vi "Build New Ballard ARINC 429 Custom Device.vi"() -> ()   [LabVIEW 2020, in "Ballard ARINC 429 Scripting Examples.lvlib"]
uses:
  Ballard ARINC 429 Scripting Examples.lvlib
  <vilib>/addons/VeriStand Custom Device Scripting APIs/Ballard ARINC 429/Custom Device Support/Shared/Direction.ctl
  <vilib>/addons/VeriStand Custom Device Scripting APIs/Ballard ARINC 429/Custom Device Support/Shared/SDI.ctl
  <vilib>/addons/VeriStand Custom Device Scripting APIs/Ballard ARINC 429/Custom Device Support/Shared/Transfer Type.ctl
  <vilib>/addons/VeriStand Custom Device Scripting APIs/Ballard ARINC 429/Custom Device Support/Shared/Parameter Definition.ctl
  <vilib>/addons/VeriStand Custom Device Scripting APIs/Ballard ARINC 429/Encoding and Decoding/Encoding.ctl
  NationalInstruments.VeriStand.SystemDefinitionAPI
  niveristand-routing-and-faulting-custom-device/Source/Scripting Examples/SLSC Switch Examples.lvlib
  <vilib>/addons/VeriStand Custom Device Scripting APIs/Ballard ARINC 429/Custom Device Support/Scripting/Ballard/Ballard ARINC 429 Scripting.lvlib
  <vilib>/addons/VeriStand Custom Device Scripting APIs/Ballard ARINC 429/Encoding and Decoding/Encoding and Decoding.lvlib
panel:
  in  "Base System Definition File":path=path "Support/Base.nivssdf"
  in  "Output System Definition File":path=path "Support/Scripted Ballard ARINC 429.nivssdf"
  in  "Hardware Configuration File":path=path "Support/HW_Rx00_Tx24_Scheduled and Dynamic Labels.xml"
  # "Overview: Demonstrates using the Ballard ARINC 429 scripting API to configure the custom device by building from configuration clusters. \n\nInstructions:\n1. Specify the Hardware Configuration File. The hardware configuration file must be consistent with the schema installed by the Ballard hardware driver at C:\\Program Files (x86)\\Astronics Ballard Technology LabVIEW Driver\\Help\\index.html. The hardware configuration file must also be consistent with the configuration in this example VI.\n2. (VeriStand) Optionally, you may open the Output System Definition File in VeriStand, configure the Target, and deploy the scripted system definition to perform avionics bus communications with Ballard ARINC 429 hardware."
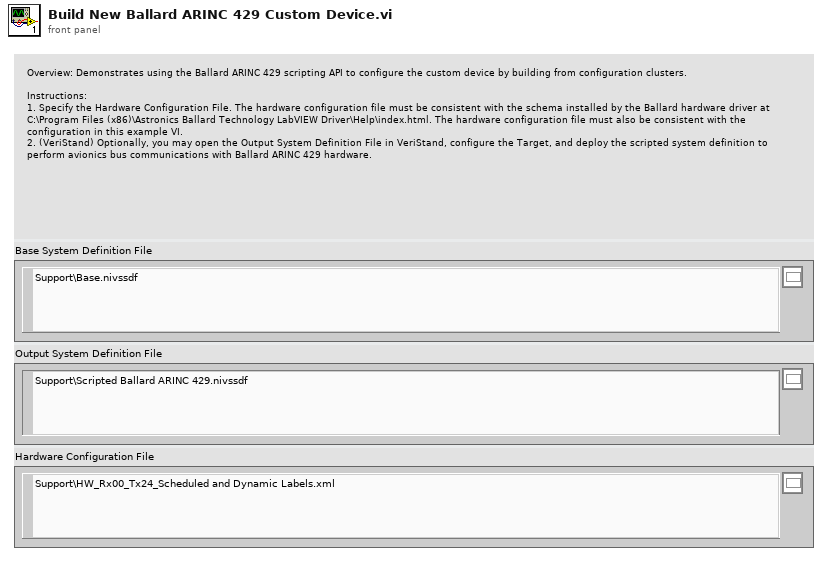
[diagram p1: front panel]
types:
  T1 = cluster{"name":string, "unit":string, "default value":dbl}[]
  T2 = typedef "Parameter Definition.ctl" = cluster{"start index":i32, "size":i32, "encoding":T3, "signed":bool, "scale multiplier":dbl, "scale offset":dbl}
  T3 = typedef "Encoding and Decoding.lvlib/Encoding.ctl" = enum16{"BNR", "BCD", "Discrete"}
  T4 = typedef "Direction.ctl" = enum16{"Rx", "Tx"}
  T5 = typedef "Transfer Type.ctl" = enum16{"Scheduled", "Acyclic", "Block", "Strobe"}
  T6 = typedef "SDI.ctl" = i32
  T7 = typedef "Custom Device API.lvlib/Custom Device Item Ref.ctl" = u64
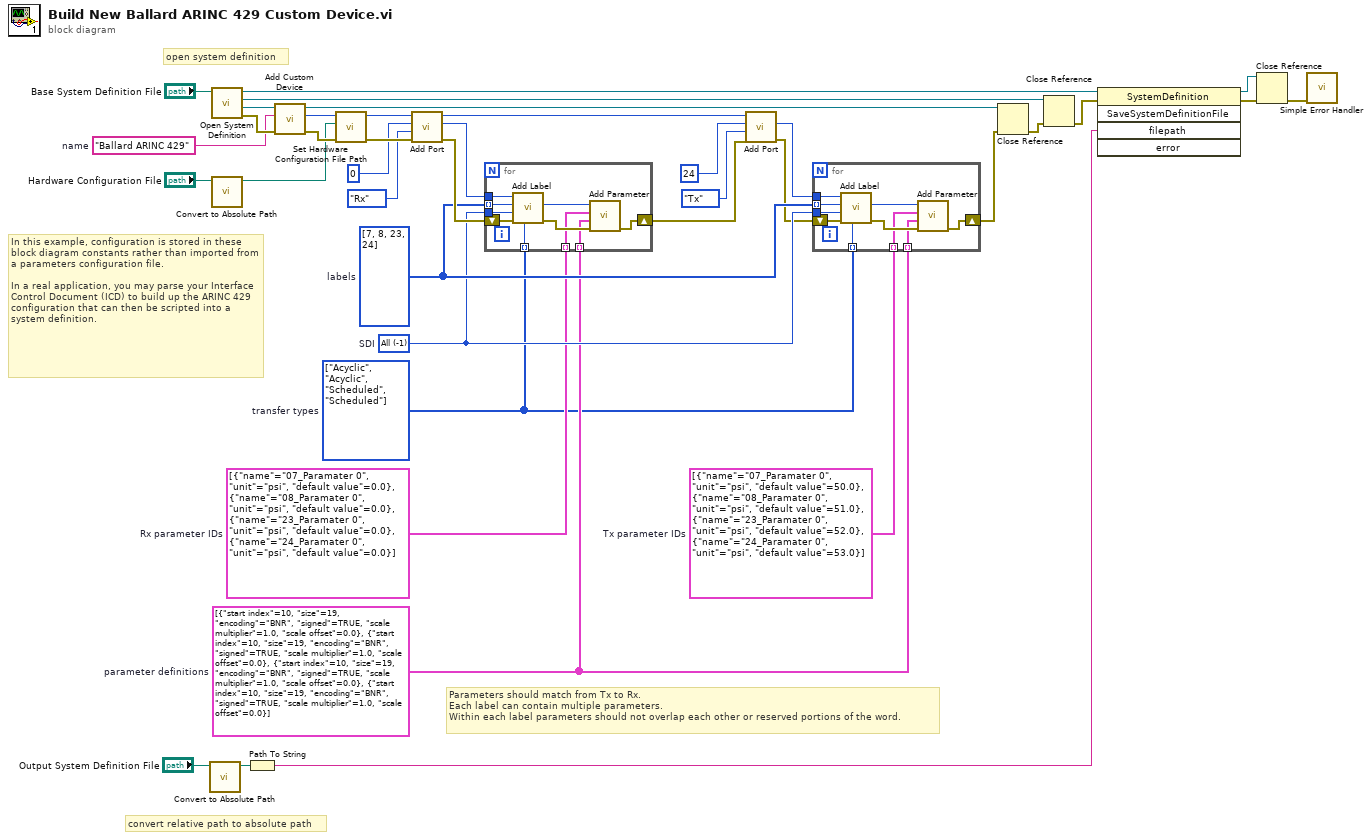
[diagram p0: block diagram]
diagram:
  w1 = T1 [{"name"="07_Paramater 0", "unit"="psi", "default value"=50.0}, {"name"="08_Paramater 0", "unit"="psi", "default value"=51.0}, {"name"="23_Paramater 0", "unit"="psi", "default value"=52.0}, {"name"="24_Paramater 0", "unit"="psi", "default value"=53.0}]  # Tx parameter IDs
  w4 = T2[] [{"start index"=10, "size"=19, "encoding"=enum."BNR", "signed"=TRUE, "scale multiplier"=1.0, "scale offset"=0.0}, {"start index"=10, "size"=19, "encoding"=enum."BNR", "signed"=TRUE, "scale multiplier"=1.0, "scale offset"=0.0}, {"start index"=10, "size"=19, "encoding"=enum."BNR", "signed"=TRUE, "scale multiplier"=1.0, "scale offset"=0.0}, {"start index"=10, "size"=19, "encoding"=enum."BNR", "signed"=TRUE, "scale multiplier"=1.0, "scale offset"=0.0}]  # parameter definitions
  w5 = T1 [{"name"="07_Paramater 0", "unit"="psi", "default value"=0.0}, {"name"="08_Paramater 0", "unit"="psi", "default value"=0.0}, {"name"="23_Paramater 0", "unit"="psi", "default value"=0.0}, {"name"="24_Paramater 0", "unit"="psi", "default value"=0.0}]  # Rx parameter IDs
  w2 = T5[] [enum."Acyclic", enum."Acyclic", enum."Scheduled", enum."Scheduled"] items=["Scheduled", "Acyclic", "Block", "Strobe"]  # transfer types
  w7 = T6 -1 items=["All"=-1, "0 (b00)"=0, "1 (b01)"=1, "2 (b10)"=2, "3 (b11)"=3]  # SDI
  w8 = u32[] [7, 8, 23, 24]  # labels
  w23 = "Ballard ARINC 429"  # name
  # "open system definition"
  # "convert relative path to absolute path"
  # "Parameters should match from Tx to Rx.\nEach label can contain multiple parameters.\nWithin each label parameters should not overlap each other or reserved portions of the word."
  # "In this example, configuration is stored in these block diagram constants rather than imported from a parameters configuration file.\n\nIn a real application, you may parse your Interface Control Document (ICD) to build up the ARINC 429 configuration that can then be scripted into a system definition."
  # "8."
  n1 = call "Convert to Absolute Path.vi"("System Definition File"="Output System Definition File") -> ("Absolute Path"=w32:path)  [unwired: 10 in]
  n2 = call "Open System Definition.vi"("System Definition File"="Base System Definition File") -> ("error out"=w26:errorcluster, "Target Refnum"=w25:refnum<k24>, "Root Refnum"=w29:refnum<k24>, "System Definition Refnum"=w30:refnum<k24>)  [unwired: 7 in]
  n3 = call "Convert to Absolute Path.vi"("System Definition File"="Hardware Configuration File") -> ("Absolute Path"=w20:path)  [unwired: 10 in]
  n4 = Path To String(path=w32) -> (string=w37:string)
  n5 = call <vilib>:"Add Custom Device.vi"("error in"=w26, "name"=w23, "target in"=w25) -> ("error out"=w21:errorcluster, "Ballard ARINC 429 ref out"=w22:T7, "target out"=w24:refnum<k24>)  [unwired: 6 in]
  n6 = call <vilib>:"Set Hardware Configuration File Path.vi"("error in"=w21, "path"=w20, "custom device ref"=w22) -> ("error out"=w18:errorcluster, "custom device ref out"=w19:T7)  [unwired: 7 in]
  n7 = call <vilib>:"Add Port.vi"("error in"=w18, "direction"=Direction."Rx", "port number"=u16 0, "custom device ref"=w19) -> ("error out"=w16:errorcluster, "port ref out"=w17:T7, "custom device ref out"=w11:T7)  [unwired: 5 in]
  n8 = for {
    tunnel: w17 -> [w48]
    tunnel: w7 -> [w46]
    shift-right: [w42] -> w10
    shift-left: w16 -> [w47]
    tunnel: w8 -> [w43] mode=indexing
    tunnel: w5 -> [w41] mode=indexing
    tunnel: w4 -> [w40] mode=indexing
    tunnel: w2 -> [w39] mode=indexing
    n9 = call <vilib>:"Add Label.vi"("transfer type"=w39, "error in"=w47, "SDI value"=w46, "label value"=w43, "port ref"=w48) -> ("error out"=w44:errorcluster, "label ref"=w45:T7)  [unwired: 4 in, 1 out]
    n10 = call <vilib>:"Add Parameter.vi"("error in"=w44, "parameter definition"=w40, "parameter"=w41, "label ref"=w45) -> ("error out"=w42:errorcluster)  [unwired: 5 in, 2 out]
  }
  n11 = call <vilib>:"Add Port.vi"("error in"=w10, "direction"=Direction."Tx", "port number"=u16 24, "custom device ref"=w11) -> ("error out"=w6:errorcluster, "port ref out"=w9:T7)  [unwired: 5 in, 1 out]
  n12 = for {
    tunnel: w9 -> [w58]
    tunnel: w7 -> [w56]
    shift-right: [w52] -> w3
    shift-left: w6 -> [w57]
    tunnel: w8 -> [w53] mode=indexing
    tunnel: w1 -> [w51] mode=indexing
    tunnel: w4 -> [w50] mode=indexing
    tunnel: w2 -> [w49] mode=indexing
    n13 = call <vilib>:"Add Label.vi"("transfer type"=w49, "error in"=w57, "SDI value"=w56, "label value"=w53, "port ref"=w58) -> ("error out"=w54:errorcluster, "label ref"=w55:T7)  [unwired: 4 in, 1 out]
    n14 = call <vilib>:"Add Parameter.vi"("error in"=w54, "parameter definition"=w50, "parameter"=w51, "label ref"=w55) -> ("error out"=w52:errorcluster)  [unwired: 5 in, 2 out]
  }
  n15 = Close Reference(reference=w24, error in (no error)=w3) -> (error out=w28:errorcluster)
  n16 = Close Reference(reference=w29, error in (no error)=w28) -> (error out=w34:errorcluster)
  n17 = invoke class="SystemDefinition" method="SaveSystemDefinitionFile"(reference=w30, error in=w34, "filepath"=w37) -> (reference out=w35:refnum<k24>, error out=w36:errorcluster)  [unwired: 2 in, 3 out]
  n18 = Close Reference(reference=w35, error in (no error)=w36) -> (error out=w33:errorcluster)
  n19 = call <vilib>:"Simple Error Handler.vi"("error in (no error)"=w33) -> ()  [unwired: 1 in, 8 out]
